vi "provide_note_book_info.vi"(8 "error in (no error)":errorcluster, 10 "notebook string in":string, 11 "DataCollectionDL091104Scaffold in":refnum<class "DataCollectionDL091104Scaffold.lvclass">) -> (0 "error out":errorcluster, 2 "notebook string out":string, 3 "DataCollectionDL091104Scaffold out":refnum<class "DataCollectionDL091104Scaffold.lvclass">)   [LabVIEW 2010, in "DataCollectionDL091104Scaffold.lvclass"]
uses:
  DataCollectionDL091104Scaffold.lvclass
  GenericDataCollection/GenericDataCollection/GenericDataCollection.lvclass
  DataCollectionDL091104Scaffold.lvclass/DataCollectionDL091104Scaffold.ctl
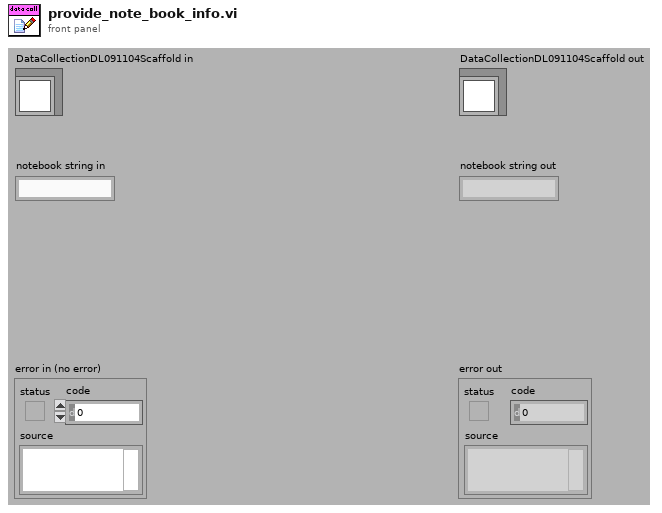
[diagram p1: front panel]
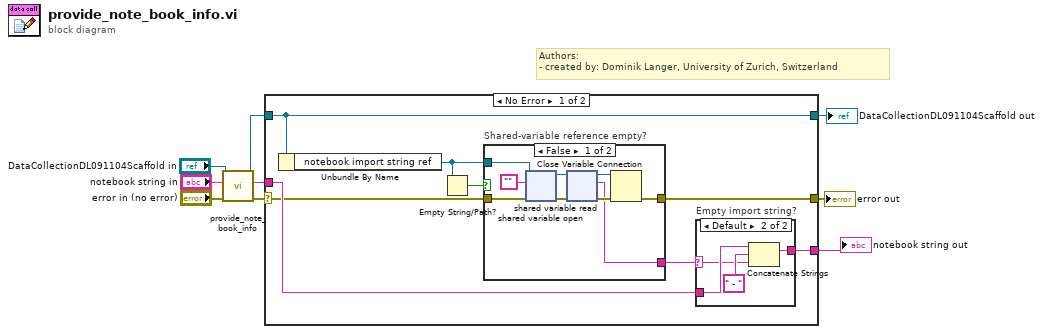
[diagram p0: block diagram]
diagram:
  # "Authors: \n- created by: Dominik Langer, University of Zurich, Switzerland"
  n1 = call-parent "provide_note_book_info.vi"("error in (no error)"="error in (no error)", "notebook string in"="notebook string in", "GenericDataCollection in"="DataCollectionDL091104Scaffold in") -> ("error out"=w6:errorcluster, "notebook string out"=w3:string, "GenericDataCollection out"=w5:refnum<class "DataCollectionDL091104Scaffold.lvclass">)  [unwired: 6 in]
  n2 = case shown="No Error" w6 {
    selector: w6 -> [w14 w33]
    tunnel: w5 -> [w17 w35]
    tunnel: [w17 w35] -> w4
    tunnel: w3 -> [w16 w34]
    tunnel: [w15 w34] -> w2
    tunnel: [w12 w33] -> w1
    frame No Error {
      n3 = Unbundle By Name(w17) -> ("notebook import string ref"=w11:refnum<k21>)
      n4 = Empty String/Path?(string/path=w11) -> (empty?=w10:bool)
      n5 = case "Shared-variable reference empty?" shown="False" w10 {
        tunnel: w14 -> [w26 w27]
        tunnel: w11 -> [w25 _]
        tunnel: [w19 _] -> w13
        tunnel: [w18 w27] -> w12
        frame False {
          n6 = shared-variable-open(w25, w26, "") -> (w23:refnum<k21>, w24:errorcluster)  [unwired: 1 in]
          n7 = shared-variable-read(w23, w24) -> (w20:refnum<k21>, w21:errorcluster, w19:string)  [unwired: 1 out]
          n8 = Close Variable Connection(8:w21, 11:w20) -> (0:w18:errorcluster)
        }
        frame True {
        }
      }
      n9 = case "Empty import string?" shown="Default" w13 {
        selector: w13 -> [_ w29]
        tunnel: w16 -> [w28 w32]
        tunnel: [w28 w31] -> w15
        frame "" {
          # "Empty string!"
        }
        frame Default {
          n10 = Concatenate Strings(w32, " - " ("string"), w29) -> (w31:string)
        }
      }
    }
    frame Error {
    }
  }
  "error out" <- w1
  "DataCollectionDL091104Scaffold out" <- w4
  "notebook string out" <- w2
